vi "End ClientStreamTemplate.vi"(8 "error in":errorcluster, 11 "Call ID in":T2) -> (0 "error out":errorcluster, 1 "errorDetails":T1, 2 "Response Data":cluster{"Numeric":dbl})   [LabVIEW 2024, in "Client Template.lvlib"]
uses:
  Client Template.lvlib
  9ddb346c-f848-4ec1-9569-72f30e6bd646.vi
  gRPC lv Support/grpc-lvsupport/grpc-lvsupport.lvlib
  gRPC lv Support/grpc-lvsupport/grpcId.ctl
  gRPC lv Support/grpc-lvsupport/Any.ctl
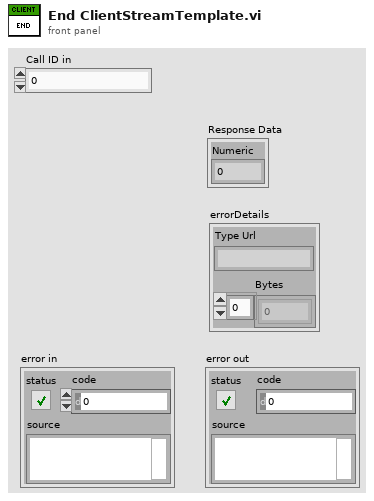
[diagram p1: front panel]
types:
  T1 = typedef "grpc-lvsupport.lvlib/Any.ctl" = cluster{"Type Url":string, "Bytes":u8[]}
  T2 = typedef "grpc-lvsupport.lvlib/grpcId.ctl" = u64
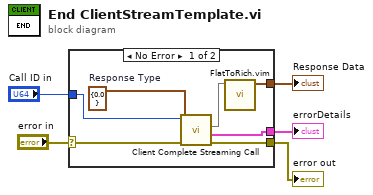
[diagram p0: block diagram]
diagram:
  n1 = case shown="No Error" "error in" {
    selector: "error in" -> [w12 w13]
    tunnel: [w11 w13] -> w4
    tunnel: "Call ID in" -> [w10 _]
    tunnel: [w6 _] -> w2
    tunnel: [w8 _] -> w1
    frame No Error {
      w9 = cluster{"Numeric":dbl} {"Numeric"=0.0}  # Response Type
      n2 = call "Client Complete Streaming Call.vi"("error in"=w12, "Cancel All Reads (F)"=w9, "Call ID in"=w10) -> ("error out"=w11:errorcluster, "errorDetails"=w8:T1, 2:w7)  [unwired: 6 in]
      n3 = call "FlatToRich.vim"("InputCluster"=w7) -> ("OutputCluster"=w6:cluster{"Numeric":dbl})  [unwired: 10 in]
    }
    frame Error {
    }
  }
  "error out" <- w4
  "Response Data" <- w2
  "errorDetails" <- w1
